vi "RSZVB Set Pulse Generator Assignment.vi"(8 "error in (no error)":errorcluster {"code" format="%.0x"}, 9 "Assignment (0)":i32(ring) items=["Gen 1 Controls All Modulators", "Gen 2 Controls All Modulators", "Gen 1 Controls Modulators 1 And 3, Gen 2 Controls Modulator 2", "Gen 1 Controls Modulators 1 And 2, Gen 2 Controls Modulator 3"], 10 "Channel (1)":i32=1, 11 "VISA session":refnum<visa-resource-name>) -> (0 "error out":errorcluster {"code" format="%.0x"}, 3 "dup VISA session":refnum<visa-resource-name>)   [LabVIEW 2011]
doc: "This VI defines the assignment between pulse generator signals and pulse modulators.\n\nRemote-control command(s):\n[SENSe<Ch>:]EUNit:PGENerator:ASSignment G1Mall | G2Mall | G1M2 | G1M3"
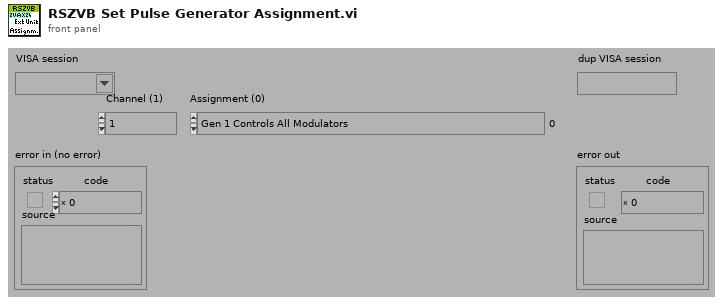
[diagram p1: front panel]
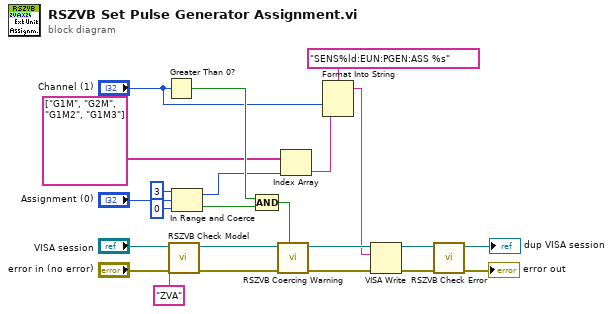
[diagram p0: block diagram]
diagram:
  n1 = Greater Than 0?(x="Channel (1)") -> (x > 0?=w12:bool)
  n2 = call "RSZVB Check Model.vi"("error in (no error)"="error in (no error)", "Model"="ZVA" ("Options"), "VISA session"="VISA session") -> ("error out"=w1:errorcluster, "dup VISA session"=w2:refnum<visa-resource-name>)  [unwired: 7 in]
  n3 = In Range and Coerce(upper limit=3, x="Assignment (0)", lower limit=0) -> (coerced(x)=w11:i32, In Range?=w13:bool)
  n4 = Compound Arithmetic op=AND(w12, w13) -> (w15:bool)
  n5 = call "RSZVB Coercing Warning.vi"("In Range?"=w15, "error in (no error)"=w1, "VISA session"=w2) -> ("error out"=w22:errorcluster, "dup VISA session"=w23:refnum<visa-resource-name>)  [unwired: 7 in]
  n6 = Index Array(array=string[] ["G1M", "G2M", "G1M2", "G1M3"], index=w11) -> (element=w10:string)
  n7 = Format Into String(format string="SENS%ld:EUN:PGEN:ASS %s", "Channel (1)", w10) -> (resulting string=w19:string)  [unwired: 2 in, 1 out]
  n8 = VISA Write(VISA resource name=w23, write buffer=w19, error in (no error)=w22) -> (VISA resource name out=w20:refnum<visa-resource-name>, error out=w21:errorcluster)  [unwired: 1 out]
  n9 = call "RSZVB Check Error.vi"("error in (no error)"=w21, "VISA session"=w20) -> ("error out"=→"error out":errorcluster, "dup VISA session"=→"dup VISA session":refnum<visa-resource-name>)  [unwired: 8 in]
